vi "PowerControl.vi"(8 "error in (no error)":errorcluster caption="错误输入（无错误）", 9 "On/Off?":bool, 10 "Addr":u8, 11 "DevControl 输入":refnum<class "DevControl.lvclass"> caption="DNL_LabVIEW Object in") -> (0 "error out":errorcluster caption="错误输出", 3 "DevControl 输出":refnum<class "DevControl.lvclass"> caption="DNL_LabVIEW Object out")   [LabVIEW 2012, in "DevControl.lvclass"]
uses:
  DevControl.lvclass
  SupportVi/DevCmd.ctl
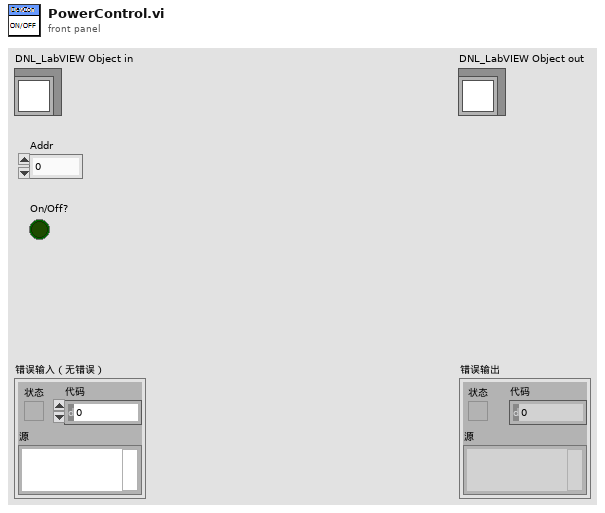
[diagram p1: front panel]
types:
  T1 = typedef "DevControl.lvclass/DevCmd.ctl" = u8
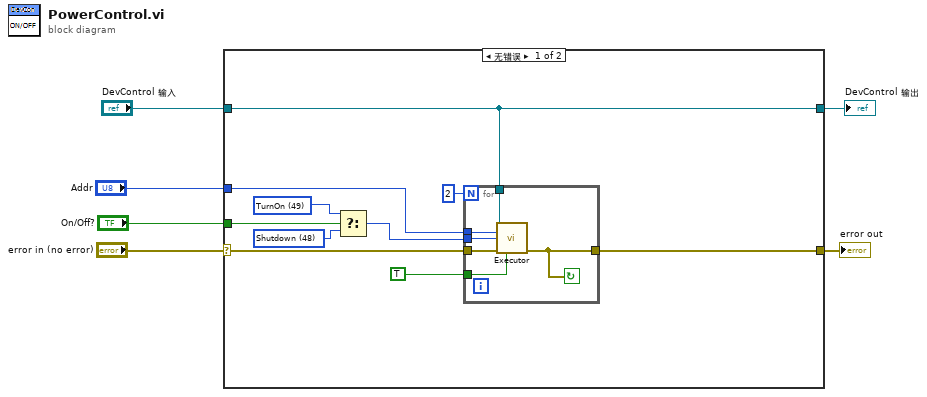
[diagram p0: block diagram]
diagram:
  n1 = case shown="无错误" "error in (no error)" {
    selector: "error in (no error)" -> [w16 w24]
    tunnel: [w8 w24] -> w5
    tunnel: [w15 w23] -> w3
    tunnel: "DevControl 输入" -> [w15 w23]
    tunnel: "Addr" -> [w14 _]
    tunnel: "On/Off?" -> [w13 _]
    frame No Error {
      w11 = T1 48 items=["WriteAddr"=81, "Enable"=80, "Red"=66, "Green"=65, "TurnOn"=49, "Shutdown"=48, "GetESD"=34] ("DevCmd")
      w12 = T1 49 items=["WriteAddr"=81, "Enable"=80, "Red"=66, "Green"=65, "TurnOn"=49, "Shutdown"=48, "GetESD"=34] ("DevCmd")
      n2 = Select(t=w12, s=w13, f=w11) -> (s? t:f=w10:T1)
      n3 = for {
        N: 2 -> [_]
        tunnel: w16 -> [w22]
        tunnel: w15 -> [w21]
        tunnel: w14 -> [w20]
        tunnel: w10 -> [w19]
        tunnel: TRUE ("ChkDat?") -> [w18]
        tunnel: [w17] -> w8
        stop <- w17 continue-if-true
        n4 = call-dynamic "Executor.vi"("DevControl 输入"=w21, "Addr"=w20, "DevCmd"=w19, "error in (no error)"=w22, "ChkDat?"=w18) -> ("error out"=w17:errorcluster)  [unwired: 8 in, 2 out]
      }
    }
    frame Error {
    }
  }
  "error out" <- w5
  "DevControl 输出" <- w3
